vi "Find Changed.vi"(8 "error in (no error)":errorcluster, 10 "Update Objects":T2={"Settings"={"Paths"=[], "Rectangles"=[], "Funnels"=[], "Dots"=[]}, "Data"={"Paths"=[], "Rectangles"=[], "SVGImage"=refnum, "Dots"=[], "Funnels"=[]}}, 11 "Tool Data in":refnum<class "Tool Data.lvclass">) -> (0 "error out":errorcluster, 3 "Tool Data out":refnum<class "Tool Data.lvclass">)   [LabVIEW 2019, in "Tool Data.lvclass"]
uses:
  Tool Data.lvclass
  Typedefs/PrivateEvents--Tool Data.Update Objects.ctl
  Parse/Image/SVGImage.lvclass
  Settings/Setting Database/Typedefs/PublicEvents--Setting Database.PathsUpdated.ctl
  Settings/Setting Database/Typedefs/PublicEvents--Setting Database.RectanglesUpdated.ctl
  Settings/Setting Database/Typedefs/PublicEvents--Setting Database.FunnelsUpdated.ctl
  Settings/Funnel Settings/Funnel Settings.lvclass
  Settings/Setting Database/Typedefs/PublicEvents--Setting Database.DotsUpdated.ctl
  Settings/Dot Settings/Dot Settings.lvclass
  Parse/Dot/Dot.lvclass
  Tool Data.lvclass/Tool Data.ctl
  Parse/ParsePaths/Path.lvclass
  Settings/Path Settings/Path Settings.lvclass
  Settings/Setting Database/Setting Database.lvclass
  Settings/Rectangle Settings/Rectangle Settings.lvclass
  Parse/Rectangle/Rectangle.lvclass
panel:
  out "Changed Objects":T1
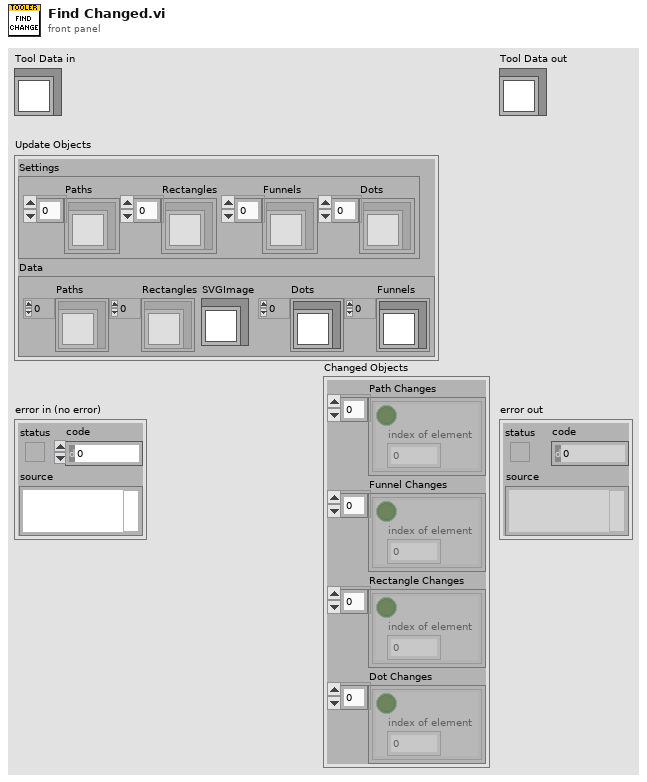
[diagram p1: front panel]
types:
  T1 = cluster{"Path Changes":cluster{bool, "index of element":i32}[], "Funnel Changes":cluster{bool, "index of element":i32}[], "Rectangle Changes":cluster{bool, "index of element":i32}[], "Dot Changes":cluster{bool, "index of element":i32}[]}
  T2 = typedef "Tool Data.lvclass/PrivateEvents--Tool Data.Update Objects.ctl" = cluster{"Settings":cluster{"Paths":T3, "Rectangles":T4, "Funnels":T5, "Dots":T6}, "Data":cluster{"Paths":refnum<class "Path.lvclass">[], "Rectangles":refnum<class "Rectangle.lvclass">[], "SVGImage":refnum<class "SVGImage.lvclass">, "Dots":refnum<class "Dot.lvclass">[], "Funnels":refnum<class "Path.lvclass">[]}}
  T3 = typedef "Setting Database.lvclass/PublicEvents--Setting Database.PathsUpdated.ctl" = refnum<class "Path Settings.lvclass">[]
  T4 = typedef "Setting Database.lvclass/PublicEvents--Setting Database.RectanglesUpdated.ctl" = refnum<class "Rectangle Settings.lvclass">[]
  T5 = typedef "Setting Database.lvclass/PublicEvents--Setting Database.FunnelsUpdated.ctl" = refnum<class "Funnel Settings.lvclass">[]
  T6 = typedef "Setting Database.lvclass/PublicEvents--Setting Database.DotsUpdated.ctl" = refnum<class "Dot Settings.lvclass">[]
  T7 = cluster{"Paths":T3, "Rectangles":T4, "Funnels":T5, "Dots":T6}
  T8 = cluster{"Paths":refnum<class "Path.lvclass">[], "Rectangles":refnum<class "Rectangle.lvclass">[], "SVGImage":refnum<class "SVGImage.lvclass">, "Dots":refnum<class "Dot.lvclass">[], "Funnels":refnum<class "Path.lvclass">[]}
  T9 = cluster{"paths":string[], "funnels":string[], "rects":string[], "dots":string[]}
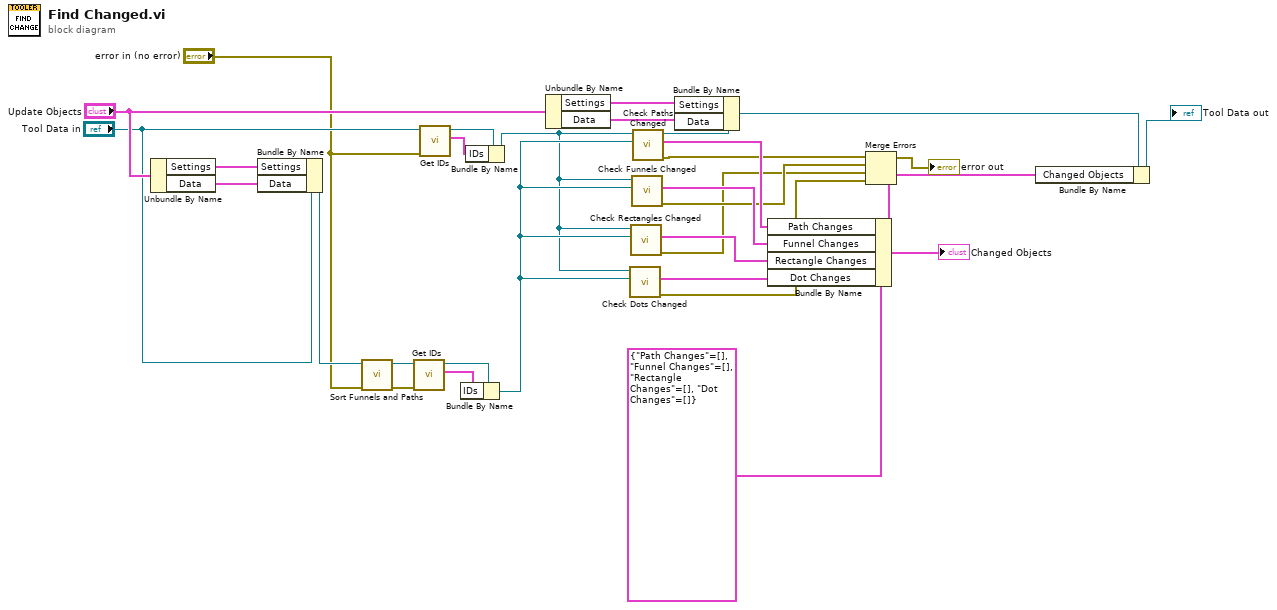
[diagram p0: block diagram]
diagram:
  n1 = Unbundle By Name("Update Objects") -> ("Settings"=w27:T7, "Data"=w26:T8)
  n2 = Bundle By Name(cluster="Tool Data in", "Settings"=w27, "Data"=w26) -> (w30:refnum<class "Tool Data.lvclass">)
  n3 = call "Sort Funnels and Paths.vi"("error in (no error)"="error in (no error)", "Tool Data in"=w30) -> ("error out"=w29:errorcluster, "Tool Data out"=w28:refnum<class "Tool Data.lvclass">)  [unwired: 8 in]
  n4 = call "Get IDs.vi"("error in (no error)"=w29, "Tool Data in"=w28) -> ("IDs"=w21:T9, "Tool Data out"=w20:refnum<class "Tool Data.lvclass">)  [unwired: 7 in, 1 out]
  n5 = call "Get IDs.vi"("error in (no error)"="error in (no error)", "Tool Data in"="Tool Data in") -> ("IDs"=w18:T9, "Tool Data out"=w19:refnum<class "Tool Data.lvclass">)  [unwired: 7 in, 1 out]
  n6 = Bundle By Name(cluster=w20, "IDs"=w21) -> (w17:refnum<class "Tool Data.lvclass">)
  n7 = Bundle By Name(cluster=w19, "IDs"=w18) -> (w16:refnum<class "Tool Data.lvclass">)
  n8 = Unbundle By Name("Update Objects") -> ("Settings"=w24:T7, "Data"=w23:T8)
  n9 = call "Check Dots Changed.vi"("New Tool"=w17, "Tool Data in"=w16) -> ("error out"=w5:errorcluster, "Changed"=w15:cluster{bool, "index of element":i32}[])  [unwired: 7 in, 1 out]
  n10 = call "Check Rectangles Changed.vi"("New Tool"=w17, "Tool Data in"=w16) -> ("error out"=w6:errorcluster, "Changed"=w13:cluster{bool, "index of element":i32}[])  [unwired: 7 in, 1 out]
  n11 = call-dynamic "Check Funnels Changed.vi"("New Tool"=w17, "Tool Data in"=w16) -> ("error out"=w7:errorcluster, "Changed"=w12:cluster{bool, "index of element":i32}[])  [unwired: 7 in, 1 out]
  n12 = call-dynamic "Check Paths Changed.vi"("New Data In"=w17, "Tool Data in"=w16) -> ("error out"=w8:errorcluster, "Changed"=w11:cluster{bool, "index of element":i32}[], "Tool Data out"=w10:refnum<class "Tool Data.lvclass">)  [unwired: 7 in]
  n13 = Bundle By Name(cluster=w10, "Settings"=w24, "Data"=w23) -> (w3:refnum<class "Tool Data.lvclass">)
  n14 = Bundle By Name(cluster=T1 {"Path Changes"=[], "Funnel Changes"=[], "Rectangle Changes"=[], "Dot Changes"=[]}, "Path Changes"=w11, "Funnel Changes"=w12, "Rectangle Changes"=w13, "Dot Changes"=w15) -> (w1:T1)
  "Changed Objects" <- w1
  n15 = Merge Errors(w8, w7, w6, w5) -> (→"error out":errorcluster)
  n16 = Bundle By Name(cluster=w3, "Changed Objects"=w1) -> (→"Tool Data out":refnum<class "Tool Data.lvclass">)
